vi "Set Server gRPC UEs.vi"(10 "Server gRPC UEs":T1, 11 "OOP Server in":refnum<class "Query Server.lvclass">) -> (3 "OOP Server out":refnum<class "Query Server.lvclass">)   [LabVIEW 2019, in "Query Server.lvlib" / "Query Server.lvclass"]
uses:
  Query Server.lvclass
  typeDefs/Server gRPC UEs.ctl
  gRPC lvSupport/Server API/typeDefs/Generic Method Event Data.ctl
  gRPC lvSupport/Server API/typeDefs/grpcId.ctl
  Query Server.lvclass/Query Server.ctl
  gRPC lvSupport/gprc-lvsupport.lvlib
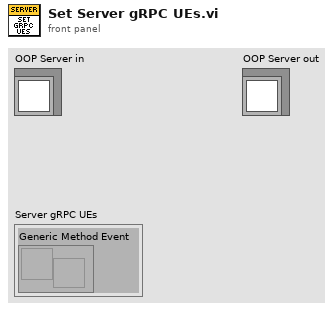
[diagram p1: front panel]
types:
  T1 = typedef "Query Server.lvlib/Query Server.lvclass/Server gRPC UEs.ctl" = cluster{"Generic Method Event":refnum<user-event>}
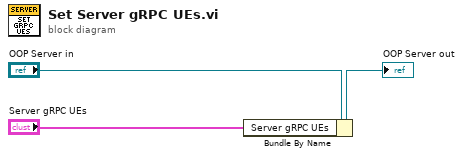
[diagram p0: block diagram]
diagram:
  n1 = Bundle By Name(cluster="OOP Server in", "Server gRPC UEs"="Server gRPC UEs") -> (→"OOP Server out":refnum<class "Query Server.lvclass">)
